vi "Create IO Channels.vi"(6 "AI Buffer Size (s)":i32=10, 7 "Num. of Cards":i32=2, 8 "AI Block Size":i32=5000, 9 "OSC Configuration":T3(array[cluster])=[[{"Signal Type"=enum."Sine Wave", "DC"=0.0, "Amplitude"=0.01, "frequency"=2.0, "Phase"=0.0}, {"Signal Type"=enum."Sine Wave", "DC"=0.001, "Amplitude"=0.005, "frequency"=2.0, "Phase"=0.0}]] {"frequency" step=0.001 format="%.3p"; "Amplitude" format="%0.2p"; "DC" min=-0.99 max=0.99 format="%.2p"}, 10 "AO Configuration":T1(array[cluster])=[{"Output physical channels"="PXI1Slot2/ao0", "AO. Max"=0.1, "AO.Min"=-0.1}, {"Output physical channels"="", "AO. Max"=0.1, "AO.Min"=-0.1}], 11 "AI Configuration":T2(array[cluster])=[{"AI.Coupling"=10050, "AI.Max"=10.0, "AI.Min"=-10.0, "Input physical channels"="PXI1Slot2/ai0:1"}, {"AI.Coupling"=10050, "AI.Max"=10.0, "AI.Min"=-10.0, "Input physical channels"="PXI1Slot3/ai0:3"}, {"AI.Coupling"=10050, "AI.Max"=10.0, "AI.Min"=-10.0, "Input physical channels"=""}] {"AI.Coupling" items=["AC"=10045, "DC"=10050, "GND"=10066]}) -> (0 "Sampling information":cluster{"Fs":dbl, "#s":dbl}[](array[cluster])=[{"Fs"=10000.0, "#s"=5000.0}, {"Fs"=10000.0, "#s"=5000.0}], 1 "AI Rate":dbl=10000.0 format="%.2f", 2 "AO Task":refnum<k21>[](array[refnum]), 3 "AI task":refnum<k21>[](array[refnum]), 4 "phase log":dbl[](array[numeric])=[0.99999999999938, 0.99999999999938])   [LabVIEW 2011, in "Lock-In Variable Channels_2.lvclass"]
uses:
  Variable Channel O.O.P/Lock-In Variable Channels_2.lvclass
  <vilib>/DAQmx/write.llb/DAQmx Write (Analog 1D Wfm NChan NSamp).vi
  <vilib>/DAQmx/create/channels.llb/DAQmx Create Channel (AI-Voltage-Basic).vi
  <vilib>/DAQmx/configure/timing.llb/DAQmx Timing (Sample Clock).vi
  DAQ-Lockin-SubVI/Lock-in Globles Multiple Inputs and Outputs.vi
  <vilib>/DAQmx/create/channels.llb/DAQmx Create Channel (AO-Voltage-Basic).vi
  <vilib>/DAQmx/configure/trigger.llb/DAQmx Start Trigger (Digital Edge).vi
  <vilib>/DAQmx/miscellaneous.llb/DAQmx Fill In Error Info.vi
  Program Files/National Instruments/LabVIEW 2011/resource/objmgr/daqmx.rc
  <vilib>/measure/NI_MABase.lvlib
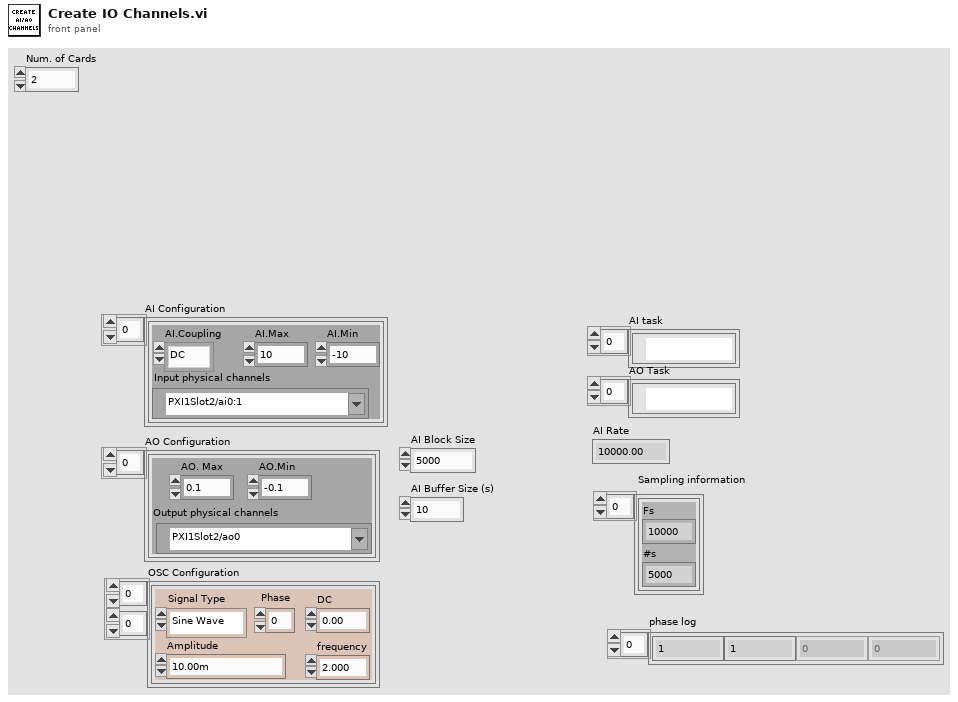
[diagram p1: front panel]
types:
  T1 = cluster{"Output physical channels":tag, "AO. Max":dbl, "AO.Min":dbl}[]
  T2 = cluster{"AI.Coupling":i32, "AI.Max":dbl, "AI.Min":dbl, "Input physical channels":tag}[]
  T3 = cluster{"Signal Type":enum16{"Sine Wave", "Triangle Wave", "Square Wave", "Sawtooth Wave"}, "DC":dbl, "Amplitude":dbl, "frequency":dbl, "Phase":dbl}[][]
  T4 = cluster{"AI.Coupling":i32, "AI.Max":dbl, "AI.Min":dbl, "Input physical channels":tag}
  T5 = cluster{"Signal Type":enum16{"Sine Wave", "Triangle Wave", "Square Wave", "Sawtooth Wave"}, "DC":dbl, "Amplitude":dbl, "frequency":dbl, "Phase":dbl}
  T6 = enum16{"Sine Wave", "Triangle Wave", "Square Wave", "Sawtooth Wave"}
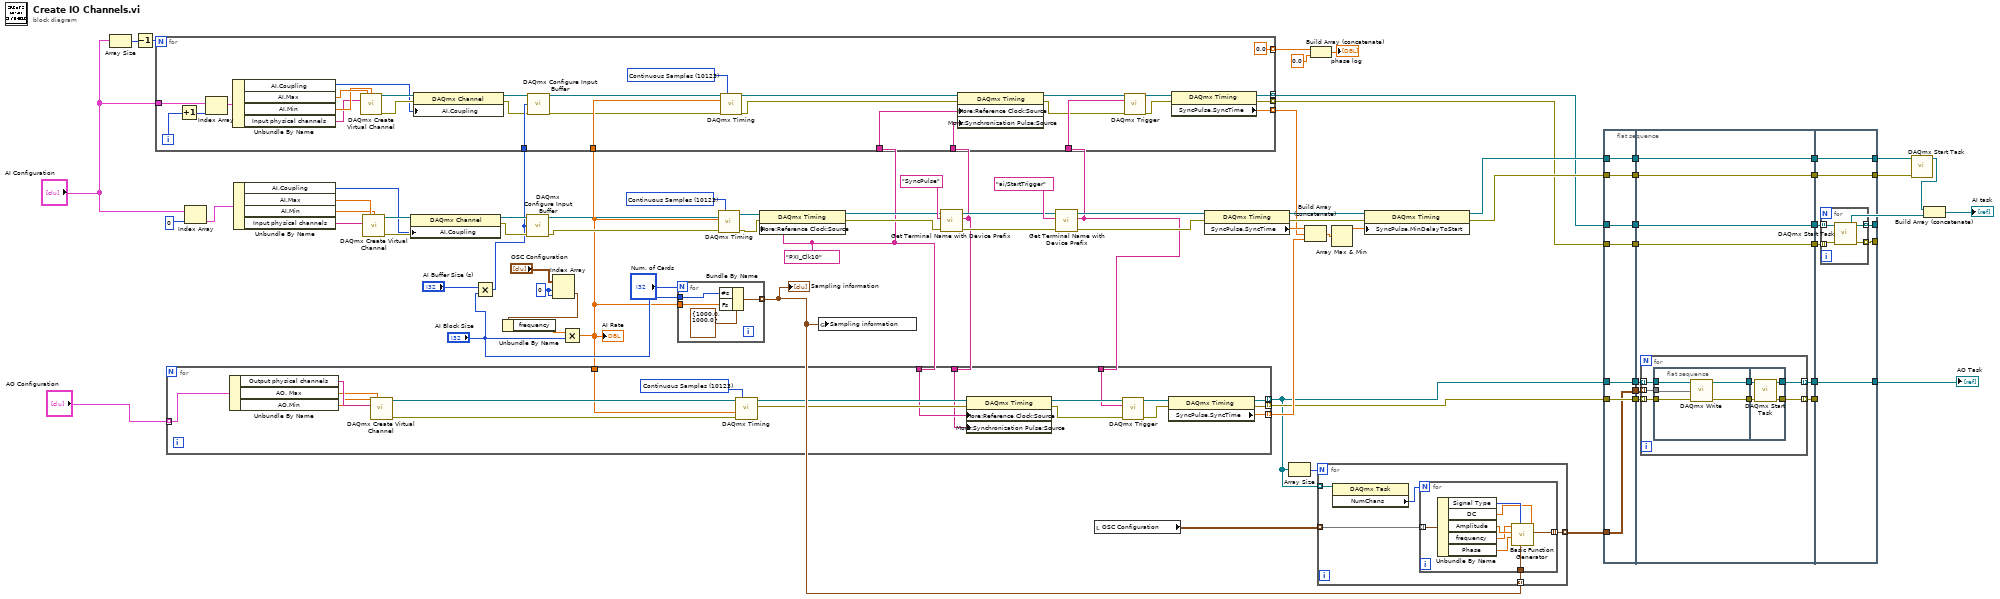
[diagram p0: block diagram]
diagram:
  w15 = 0 ("index (row)")
  w13 = tag "PXI_Clk10" ("RefClk.Src")
  w63 = 10123 items=["Finite Samples"=10178, "Continuous Samples"=10123] ("sample mode")
  n1 = Array Size(array="AI Configuration") -> (size(s)=w18:i32)
  n2 = Decrement(x=w18) -> (x-1=w17:i32)
  n3 = Index Array(array="AI Configuration", index=0) -> (element=w64:T4)
  n4 = Unbundle By Name(w64) -> ("AI.Coupling"=w36:i32, "AI.Max"=w43:dbl, "AI.Min"=w42:dbl, "Input physical channels"=w44:tag)
  n5 = call-poly <vilib>:"DAQmx Create Virtual Channel.vi"("maximum value"=w43, "minimum value"=w42, "physical channels"=w44) -> ("task out"=w38:refnum<k21>, "error out"=w37:errorcluster)  [unwired: 11 in]
  n6 = property class="DAQmx Channel"(reference=w38, error in=w37, "AI.Coupling"=w36) -> (reference out=w35:refnum<k21>, error out=w34:errorcluster)
  n7 = Multiply(x="AI Buffer Size (s)", y="AI Block Size") -> (x*y=w16:i32)
  n8 = call <vilib>:"DAQmx Configure Input Buffer.vi"("task/channels in"=w35, "buffer size (in samples per channel)"=w16, "error in"=w34) -> ("task out"=w33:refnum<k21>, "error out"=w32:errorcluster)  [unwired: 11 in]
  n9 = Index Array(array="OSC Configuration", index (row)=w15, index (col)=w15) -> (element=w26:T5)
  n10 = Unbundle By Name(w26) -> ("frequency"=w25:dbl)
  n11 = Multiply(x=w25, y="AI Block Size") -> (x*y=w14:dbl)
  "AI Rate" <- w14
  n12 = for {
    N: "Num. of Cards" -> [_]
    tunnel: w14 -> [w82]
    tunnel: "AI Block Size" -> [w81]
    tunnel: [w79] -> w4 mode=indexing
    n13 = Bundle By Name(cluster=cluster{"Fs":dbl, "#s":dbl} {"Fs"=1000.0, "#s"=1000.0} ("sampling info"), "#s"=w81, "Fs"=w82) -> (w79:cluster{"Fs":dbl, "#s":dbl})
  }
  "Sampling information" <- w4
  n14 = call-poly <vilib>:"DAQmx Timing.vi"("task/channels in"=w33, "sample mode"=w63, "rate"=w14, "error in"=w32) -> ("task out"=w62:refnum<k21>, "error out"=w61:errorcluster)  [unwired: 10 in]
  n15 = property class="DAQmx Timing"(reference=w62, error in=w61, "More:Reference Clock:Source"=w13) -> (reference out=w40:refnum<k21>, error out=w39:errorcluster)
  n16 = global write "Lock-in Globles Multiple Inputs and Outputs.vi" "Sampling information"(w4) -> ()
  n17 = call "Get Terminal Name with Device Prefix.vi"("error in (no error)"=w39, "Local Terminal Name"="SyncPulse", "task/channels in"=w40) -> ("error out"=w56:errorcluster, "Terminal Name with Device Prefix"=w12:tag, "task out"=w57:refnum<k21>)  [unwired: 6 in]
  n18 = call "Get Terminal Name with Device Prefix.vi"("error in (no error)"=w56, "Local Terminal Name"="ai/StartTrigger", "task/channels in"=w57) -> ("error out"=w54:errorcluster, "Terminal Name with Device Prefix"=w22:tag, "task out"=w55:refnum<k21>)  [unwired: 6 in]
  n19 = for {
    N: w17 -> [_]
    tunnel: "AI Configuration" -> [w110]
    tunnel: w16 -> [w112]
    tunnel: w14 -> [w111]
    tunnel: w13 -> [w109]
    tunnel: w12 -> [w108]
    tunnel: w22 -> [w107]
    tunnel: [w106] -> w21 mode=indexing
    tunnel: [w105] -> w19 mode=indexing
    tunnel: [w104] -> w20 mode=indexing
    tunnel: [0.0] -> w8 mode=indexing
    i -> [w85]
    w94 = 10123 items=["Finite Samples"=10178, "Continuous Samples"=10123, "Hardware Timed Single Point"=12522] ("sample mode")
    n20 = Increment(x=w85) -> (x+1=w84:i32)
    n21 = Index Array(array=w110, index=w84) -> (element=w93:T4)
    n22 = Unbundle By Name(w93) -> ("AI.Coupling"=w98:i32, "AI.Max"=w103:dbl, "AI.Min"=w102:dbl, "Input physical channels"=w101:tag)
    n23 = call-poly <vilib>:"DAQmx Create Virtual Channel.vi"("maximum value"=w103, "minimum value"=w102, "physical channels"=w101) -> ("task out"=w99:refnum<k21>, "error out"=w100:errorcluster)  [unwired: 11 in]
    n24 = property class="DAQmx Channel"(reference=w99, error in=w100, "AI.Coupling"=w98) -> (reference out=w97:refnum<k21>, error out=w96:errorcluster)
    n25 = call <vilib>:"DAQmx Configure Input Buffer.vi"("task/channels in"=w97, "buffer size (in samples per channel)"=w112, "error in"=w96) -> ("task out"=w95:refnum<k21>, "error out"=w88:errorcluster)  [unwired: 11 in]
    n26 = call-poly <vilib>:"DAQmx Timing.vi"("task/channels in"=w95, "sample mode"=w94, "rate"=w111, "error in"=w88) -> ("task out"=w92:refnum<k21>, "error out"=w87:errorcluster)  [unwired: 10 in]
    n27 = property class="DAQmx Timing"(reference=w92, error in=w87, "More:Reference Clock:Source"=w109, "More:Synchronization Pulse:Source"=w108) -> (reference out=w91:refnum<k21>, error out=w86:errorcluster)
    n28 = call-poly <vilib>:"DAQmx Trigger.vi"("task/channels in"=w91, "source"=w107, "error in"=w86) -> ("task out"=w90:refnum<k21>, "error out"=w89:errorcluster)  [unwired: 11 in]
    n29 = property class="DAQmx Timing"(reference=w90, error in=w89) -> (reference out=w104:refnum<k21>, error out=w105:errorcluster, "SyncPulse.SyncTime"=w106:dbl)
  }
  n30 = for {
    tunnel: [w125] -> w48 mode=indexing
    tunnel: [w124] -> w45 mode=indexing
    tunnel: [w118] -> w5 mode=indexing
    tunnel: w22 -> [w117]
    tunnel: "AO Configuration" -> [w113] mode=indexing
    tunnel: w14 -> [w116]
    tunnel: w13 -> [w115]
    tunnel: w12 -> [w114]
    w132 = 10123 items=["Finite Samples"=10178, "Continuous Samples"=10123] ("sample mode")
    n31 = Unbundle By Name(w113) -> ("Output physical channels"=w121:tag, "AO. Max"=w120:dbl, "AO.Min"=w119:dbl)
    n32 = call-poly <vilib>:"DAQmx Create Virtual Channel.vi"("maximum value"=w120, "minimum value"=w119, "physical channels"=w121) -> ("task out"=w123:refnum<k21>, "error out"=w122:errorcluster)  [unwired: 11 in]
    n33 = call-poly <vilib>:"DAQmx Timing.vi"("task/channels in"=w123, "sample mode"=w132, "rate"=w116, "error in"=w122) -> ("task out"=w131:refnum<k21>, "error out"=w130:errorcluster)  [unwired: 10 in]
    n34 = property class="DAQmx Timing"(reference=w131, error in=w130, "More:Reference Clock:Source"=w115, "More:Synchronization Pulse:Source"=w114) -> (reference out=w129:refnum<k21>, error out=w128:errorcluster)
    n35 = call-poly <vilib>:"DAQmx Trigger.vi"("task/channels in"=w129, "source"=w117, "error in"=w128) -> ("task out"=w126:refnum<k21>, "error out"=w127:errorcluster)  [unwired: 11 in]
    n36 = property class="DAQmx Timing"(reference=w126, error in=w127) -> (reference out=w118:refnum<k21>, error out=w124:errorcluster, "SyncPulse.SyncTime"=w125:dbl)
  }
  n37 = local read "OSC Configuration"() -> (w23:T3)
  n38 = property class="DAQmx Timing"(reference=w55, error in=w54) -> (reference out=w51:refnum<k21>, error out=w52:errorcluster, "SyncPulse.SyncTime"=w53:dbl)
  n39 = Array Size(array=w5) -> (size(s)=w6:i32)
  n40 = Build Array (concatenate)(w53, w21, w48) -> (w50:dbl[])
  n41 = Build Array (concatenate)(w8, 0.0) -> (→"phase log":dbl[])
  n42 = for {
    N: w6 -> [_]
    tunnel: w23 -> [w137] mode=indexing
    tunnel: [w136] -> w11 mode=indexing
    tunnel: w5 -> [w134] mode=indexing
    tunnel: w4 -> [w133] mode=indexing
    n43 = property class="DAQmx Task"(reference=w134) -> ("NumChans"=w135:u32)  [unwired: 1 in, 2 out]
    n44 = for {
      N: w135 -> [_]
      tunnel: w137 -> [w139] mode=indexing
      tunnel: [w140] -> w136 mode=indexing
      tunnel: w133 -> [w138]
      n45 = Unbundle By Name(w139) -> ("Signal Type"=w145:T6, "DC"=w144:dbl, "Amplitude"=w143:dbl, "frequency"=w142:dbl, "Phase"=w141:dbl)
      n46 = call <vilib>:"Basic Function Generator.vi"("offset"=w144, "sampling info"=w138, "signal type"=w145, "phase"=w141, "amplitude"=w143, "frequency"=w142) -> ("signal out"=w140:waveform(dbl))  [unwired: 3 in, 2 out]
    }
  }
  n47 = Array Max & Min(array=w50) -> (max value=w49:dbl)  [unwired: 3 out]
  n48 = property class="DAQmx Timing"(reference=w51, error in=w52, "SyncPulse.MinDelayToStart"=w49) -> (reference out=w46:refnum<k21>, error out=w47:errorcluster)
  n49 = flat-sequence {
    tunnel: w47 -> [w151]
    tunnel: w46 -> [w152]
    tunnel: [w152] -> w78
    tunnel: [w151] -> w77
    tunnel: [w150] -> w76
    tunnel: w45 -> [w150]
    tunnel: [w149] -> w75
    tunnel: w5 -> [w149]
    tunnel: [w146] -> w74
    tunnel: w11 -> [w146]
    tunnel: w20 -> [w148]
    tunnel: [w148] -> w73
    tunnel: [w147] -> w72
    tunnel: w19 -> [w147]
    tunnel: [w161] -> w71
    tunnel: [w160] -> w70
    tunnel: w78 -> [w161]
    tunnel: w77 -> [w160]
    tunnel: w76 -> [w159]
    tunnel: w75 -> [w158]
    tunnel: w74 -> [w157]
    tunnel: [w156] -> w69
    tunnel: w73 -> [w156]
    tunnel: [w155] -> w68
    tunnel: w72 -> [w155]
    tunnel: [w154] -> w67
    tunnel: [w153] -> w66
    tunnel: [w183] -> _
    tunnel: [w184] -> w28
    tunnel: [w182] -> w60
    tunnel: [w181] -> w59
    tunnel: w71 -> [w182]
    tunnel: w70 -> [w181]
    tunnel: w69 -> [w180]
    tunnel: w68 -> [w179]
    tunnel: w67 -> [_]
    tunnel: [w178] -> w10
    tunnel: w66 -> [w178]
    frame #0 {
    }
    frame #1 {
      n50 = for {
        tunnel: w159 -> [w162] mode=indexing
        tunnel: w158 -> [w168] mode=indexing
        tunnel: w157 -> [w167] mode=indexing
        tunnel: [w164] -> w154 mode=indexing
        tunnel: [w163] -> w153 mode=indexing
        n51 = flat-sequence {
          tunnel: w162 -> [w173]
          tunnel: w168 -> [w172]
          tunnel: w167 -> [w169]
          tunnel: [w171] -> w166
          tunnel: [w170] -> w165
          tunnel: w166 -> [w177]
          tunnel: w165 -> [w174]
          tunnel: [w176] -> w164
          tunnel: [w175] -> w163
          frame #0 {
            n52 = call-poly <vilib>:"DAQmx Write.vi"("task/channels in"=w172, "data"=w169, "error in"=w173) -> ("task out"=w170:refnum<k21>, "error out"=w171:errorcluster)  [unwired: 10 in, 1 out]
          }
          frame #1 {
            n53 = call <vilib>:"DAQmx Start Task.vi"("task/channels in"=w174, "error in"=w177) -> ("task out"=w175:refnum<k21>, "error out"=w176:errorcluster)  [unwired: 12 in]
          }
        }
      }
    }
    frame #2 {
      n54 = for {
        tunnel: [w188] -> w184 mode=indexing
        tunnel: [w187] -> w183 mode=indexing
        tunnel: w180 -> [w186] mode=indexing
        tunnel: w179 -> [w185] mode=indexing
        n55 = call <vilib>:"DAQmx Start Task.vi"("task/channels in"=w186, "error in"=w185) -> ("task out"=w188:refnum<k21>, "error out"=w187:errorcluster)  [unwired: 12 in]
      }
    }
  }
  n56 = call <vilib>:"DAQmx Start Task.vi"("task/channels in"=w60, "error in"=w59) -> ("task out"=w29:refnum<k21>)  [unwired: 12 in, 1 out]
  n57 = Build Array (concatenate)(w29, w28) -> (→"AI task":refnum<k21>[])
  "AO Task" <- w10
